vi "Configure Report Basic.vi"(0 "VISA resource name":refnum<visa-resource-name>, 5 "Data Type":T2={"Report1 (1: Ave)"=1, "Report2 (2: Max)"=2, "Report3 (3: Min) "=3, "Report4 (4: Sum) "=4, "Report5 (5: Inst) "=5} {"Report5 (5: Inst)" items=["Off", "Ave", "Max", "Min", "Sum", "Inst"]; "Report4 (4: Sum)" items=["Off", "Ave", "Max", "Min", "Sum", "Inst"]; "Report3 (3: Min)" items=["Off", "Ave", "Max", "Min", "Sum", "Inst"]; "Report2 (2: Max)" items=["Off", "Ave", "Max", "Min", "Sum", "Inst"]; "Report1 (1: Ave)" items=["Off", "Ave", "Max", "Min", "Sum", "Inst"]}, 7 "File Type (1: Combine)":i32(ring)=1 items=["Separate", "Combine"], 9 "Report Template Output":T1, 11 "error in (no error)":errorcluster, 12 "Electronic Signature (Off)":bool, 13 "Batch Info (Off)":bool) -> (4 "VISA resource name out":refnum<visa-resource-name>, 15 "error out":errorcluster)   [LabVIEW 2020, in "Yokogawa GX Series.lvlib"]
doc: "Sets report basic.\n\nCommand: SRepData\n SRepTemp\n SDigitalSign\n SRepBatchInfo"
uses:
  <instrlib>/Yokogawa GX Series/Yokogawa GX Series.lvlib
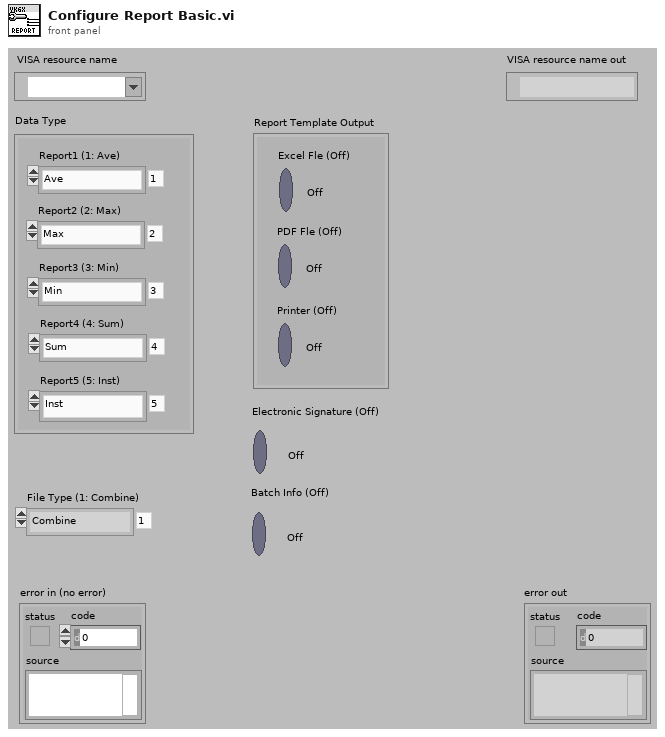
[diagram p1: front panel]
types:
  T1 = cluster{"Excel Fle (Off)":bool, "PDF Fle (Off)":bool, "Printer (Off)":bool}
  T2 = cluster{"Report1 (1: Ave)":i32, "Report2 (2: Max)":i32, "Report3 (3: Min) ":i32, "Report4 (4: Sum) ":i32, "Report5 (5: Inst) ":i32}
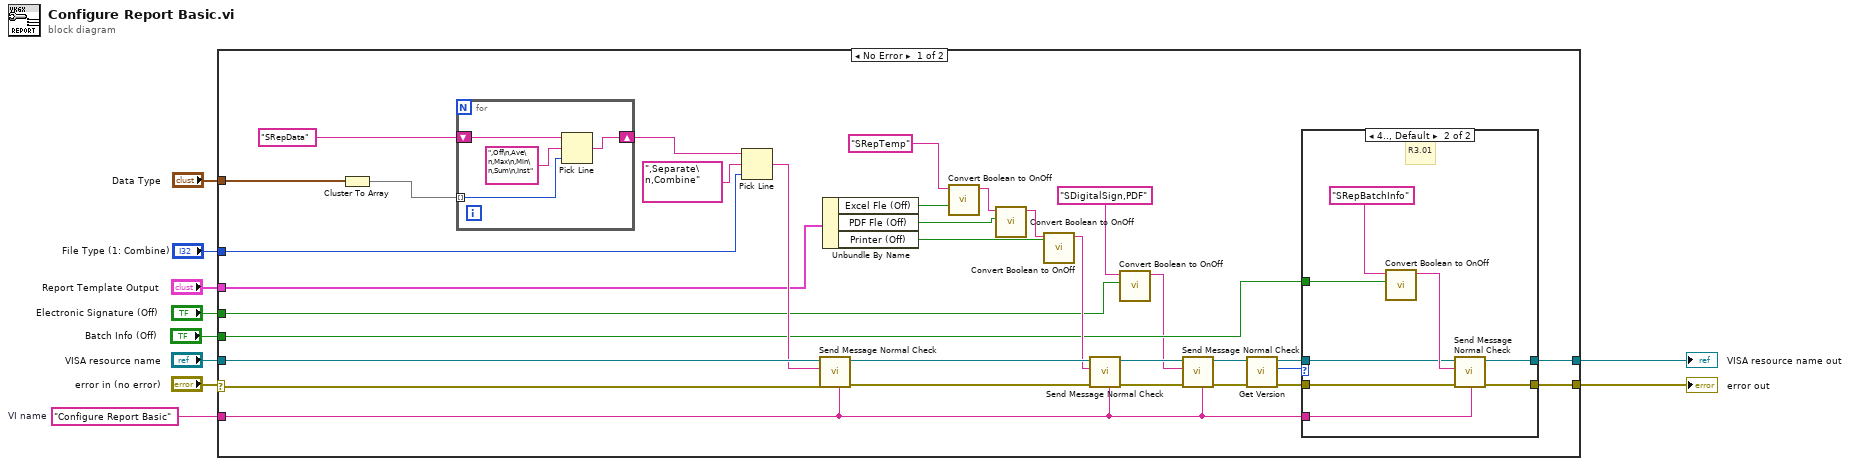
[diagram p0: block diagram]
diagram:
  w9 = "Configure Report Basic"  # VI name
  n1 = case shown="No Error" "error in (no error)" {
    selector: "error in (no error)" -> [w36 w58]
    tunnel: "VISA resource name" -> [w37 w59]
    tunnel: w9 -> [w17 _]
    tunnel: [w11 w59] -> w8
    tunnel: [w21 w58] -> w7
    tunnel: "File Type (1: Combine)" -> [w38 _]
    tunnel: "Data Type" -> [w43 _]
    tunnel: "Report Template Output" -> [w34 _]
    tunnel: "Electronic Signature (Off)" -> [w23 _]
    tunnel: "Batch Info (Off)" -> [w22 _]
    frame No Error {
      n2 = Cluster To Array(cluster=w43) -> (array=w42:i32[])
      n3 = for {
        tunnel: w42 -> [w56] mode=indexing
        shift-right: [w54] -> w40
        shift-left: "SRepData" -> [w55]
        n4 = Pick Line(string ("")=w55, multi-line string=",Off\n,Ave\n,Max\n,Min\n,Sum\n,Inst", line index=w56) -> (output string=w54:string)
      }
      n5 = Pick Line(string ("")=w40, multi-line string=",Separate\n,Combine", line index=w38) -> (output string=w35:string)
      n6 = call <instrlib>:"Send Message Normal Check.vi"("Source (\"\")"=w17, "error in (no error)"=w36, "Send Message (\"\")"=w35, "VISA resource name"=w37) -> ("error out"=w26:errorcluster, "VISA resource name out"=w27:refnum<visa-resource-name>)  [unwired: 2 in, 4 out]
      n7 = Unbundle By Name(w34) -> ("Excel Fle (Off)"=w33:bool, "PDF Fle (Off)"=w32:bool, "Printer (Off)"=w31:bool)
      n8 = call <instrlib>:"Convert Boolean to OnOff.vi"("On/Off"=w33, "Initial String (\"\")"="SRepTemp") -> ("Resulting String"=w29:string)  [unwired: 9 in]
      n9 = call <instrlib>:"Convert Boolean to OnOff.vi"("On/Off"=w32, "Initial String (\"\")"=w29) -> ("Resulting String"=w28:string)  [unwired: 9 in]
      n10 = call <instrlib>:"Convert Boolean to OnOff.vi"("On/Off"=w31, "Initial String (\"\")"=w28) -> ("Resulting String"=w25:string)  [unwired: 9 in]
      n11 = call <instrlib>:"Send Message Normal Check.vi"("Source (\"\")"=w17, "error in (no error)"=w26, "Send Message (\"\")"=w25, "VISA resource name"=w27) -> ("error out"=w19:errorcluster, "VISA resource name out"=w20:refnum<visa-resource-name>)  [unwired: 2 in, 4 out]
      n12 = call <instrlib>:"Convert Boolean to OnOff.vi"("On/Off"=w23, "Initial String (\"\")"="SDigitalSign,PDF") -> ("Resulting String"=w18:string)  [unwired: 9 in]
      n13 = call <instrlib>:"Send Message Normal Check.vi"("Source (\"\")"=w17, "error in (no error)"=w19, "Send Message (\"\")"=w18, "VISA resource name"=w20) -> ("error out"=w15:errorcluster, "VISA resource name out"=w16:refnum<visa-resource-name>)  [unwired: 2 in, 4 out]
      n14 = call <instrlib>:"Get Version.vi"("error in (no error)"=w15, "VISA resource name"=w16) -> ("error out"=w12:errorcluster, "Version"=w14:i32, "VISA resource name out"=w13:refnum<visa-resource-name>)  [unwired: 7 in]
      n15 = case shown="4.., Default" w14 {
        tunnel: w22 -> [_ w52]
        tunnel: [w44 w50] -> w11
        tunnel: [w45 w49] -> w21
        tunnel: w17 -> [_ w48]
        tunnel: w13 -> [w44 w47]
        tunnel: w12 -> [w45 w46]
        frame 0..3 {
          # "R1.03, R2.02, R2.03"
        }
        frame 4.., Default {
          # "R3.01"
          n16 = call <instrlib>:"Convert Boolean to OnOff.vi"("On/Off"=w52, "Initial String (\"\")"="SRepBatchInfo") -> ("Resulting String"=w51:string)  [unwired: 9 in]
          n17 = call <instrlib>:"Send Message Normal Check.vi"("Source (\"\")"=w48, "error in (no error)"=w46, "Send Message (\"\")"=w51, "VISA resource name"=w47) -> ("error out"=w49:errorcluster, "VISA resource name out"=w50:refnum<visa-resource-name>)  [unwired: 2 in, 4 out]
        }
      }
    }
    frame Error {
    }
  }
  "error out" <- w7
  "VISA resource name out" <- w8
